vi "Cholesky Decomposition.vi"   [LabVIEW 2020]
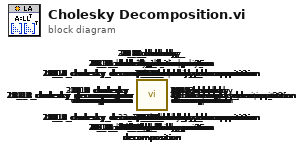
[diagram p0: block diagram]
diagram:
  n1 = call "32_16_cholesky_decomposition.vi"() -> ()  [unwired: 3 in, 1 out]
  n2 = call "32_15_cholesky_decomposition.vi"() -> ()  [unwired: 3 in, 1 out]
  n3 = call "32_14_cholesky_decomposition.vi"() -> ()  [unwired: 3 in, 1 out]
  n4 = call "32_13_cholesky_decomposition.vi"() -> ()  [unwired: 3 in, 1 out]
  n5 = call "32_12_cholesky_decomposition.vi"() -> ()  [unwired: 3 in, 1 out]
  n6 = call "32_11_cholesky_decomposition.vi"() -> ()  [unwired: 3 in, 1 out]
  n7 = call "32_10_cholesky_decomposition.vi"() -> ()  [unwired: 3 in, 1 out]
  n8 = call "32_9_cholesky_decomposition.vi"() -> ()  [unwired: 3 in, 1 out]
  n9 = call "32_8_cholesky_decomposition.vi"() -> ()  [unwired: 3 in, 1 out]
  n10 = call "32_7_cholesky_decomposition.vi"() -> ()  [unwired: 3 in, 1 out]
  n11 = call "32_6_cholesky_decomposition.vi"() -> ()  [unwired: 3 in, 1 out]
  n12 = call "32_5_cholesky_decomposition.vi"() -> ()  [unwired: 3 in, 1 out]
  n13 = call "32_4_cholesky_decomposition.vi"() -> ()  [unwired: 3 in, 1 out]
  n14 = call "32_3_cholesky_decomposition.vi"() -> ()  [unwired: 3 in, 1 out]
  n15 = call "32_2_cholesky_decomposition.vi"() -> ()  [unwired: 3 in, 1 out]
  n16 = call "32_1_cholesky_decomposition.vi"() -> ()  [unwired: 3 in, 1 out]
  n17 = call "31_16_cholesky_decomposition.vi"() -> ()  [unwired: 3 in, 1 out]
  n18 = call "31_15_cholesky_decomposition.vi"() -> ()  [unwired: 3 in, 1 out]
  n19 = call "31_14_cholesky_decomposition.vi"() -> ()  [unwired: 3 in, 1 out]
  n20 = call "31_13_cholesky_decomposition.vi"() -> ()  [unwired: 3 in, 1 out]
  n21 = call "31_12_cholesky_decomposition.vi"() -> ()  [unwired: 3 in, 1 out]
  n22 = call "31_11_cholesky_decomposition.vi"() -> ()  [unwired: 3 in, 1 out]
  n23 = call "31_10_cholesky_decomposition.vi"() -> ()  [unwired: 3 in, 1 out]
  n24 = call "31_9_cholesky_decomposition.vi"() -> ()  [unwired: 3 in, 1 out]
  n25 = call "31_8_cholesky_decomposition.vi"() -> ()  [unwired: 3 in, 1 out]
  n26 = call "31_7_cholesky_decomposition.vi"() -> ()  [unwired: 3 in, 1 out]
  n27 = call "31_6_cholesky_decomposition.vi"() -> ()  [unwired: 3 in, 1 out]
  n28 = call "31_5_cholesky_decomposition.vi"() -> ()  [unwired: 3 in, 1 out]
  n29 = call "31_4_cholesky_decomposition.vi"() -> ()  [unwired: 3 in, 1 out]
  n30 = call "31_3_cholesky_decomposition.vi"() -> ()  [unwired: 3 in, 1 out]
  n31 = call "31_2_cholesky_decomposition.vi"() -> ()  [unwired: 3 in, 1 out]
  n32 = call "31_1_cholesky_decomposition.vi"() -> ()  [unwired: 3 in, 1 out]
  n33 = call "30_16_cholesky_decomposition.vi"() -> ()  [unwired: 3 in, 1 out]
  n34 = call "30_15_cholesky_decomposition.vi"() -> ()  [unwired: 3 in, 1 out]
  n35 = call "30_14_cholesky_decomposition.vi"() -> ()  [unwired: 3 in, 1 out]
  n36 = call "30_13_cholesky_decomposition.vi"() -> ()  [unwired: 3 in, 1 out]
  n37 = call "30_12_cholesky_decomposition.vi"() -> ()  [unwired: 3 in, 1 out]
  n38 = call "30_11_cholesky_decomposition.vi"() -> ()  [unwired: 3 in, 1 out]
  n39 = call "30_10_cholesky_decomposition.vi"() -> ()  [unwired: 3 in, 1 out]
  n40 = call "30_9_cholesky_decomposition.vi"() -> ()  [unwired: 3 in, 1 out]
  n41 = call "30_8_cholesky_decomposition.vi"() -> ()  [unwired: 3 in, 1 out]
  n42 = call "30_7_cholesky_decomposition.vi"() -> ()  [unwired: 3 in, 1 out]
  n43 = call "30_6_cholesky_decomposition.vi"() -> ()  [unwired: 3 in, 1 out]
  n44 = call "30_5_cholesky_decomposition.vi"() -> ()  [unwired: 3 in, 1 out]
  n45 = call "30_4_cholesky_decomposition.vi"() -> ()  [unwired: 3 in, 1 out]
  n46 = call "30_3_cholesky_decomposition.vi"() -> ()  [unwired: 3 in, 1 out]
  n47 = call "30_2_cholesky_decomposition.vi"() -> ()  [unwired: 3 in, 1 out]
  n48 = call "30_1_cholesky_decomposition.vi"() -> ()  [unwired: 3 in, 1 out]
  n49 = call "29_16_cholesky_decomposition.vi"() -> ()  [unwired: 3 in, 1 out]
  n50 = call "29_15_cholesky_decomposition.vi"() -> ()  [unwired: 3 in, 1 out]
  n51 = call "29_14_cholesky_decomposition.vi"() -> ()  [unwired: 3 in, 1 out]
  n52 = call "29_13_cholesky_decomposition.vi"() -> ()  [unwired: 3 in, 1 out]
  n53 = call "29_12_cholesky_decomposition.vi"() -> ()  [unwired: 3 in, 1 out]
  n54 = call "29_11_cholesky_decomposition.vi"() -> ()  [unwired: 3 in, 1 out]
  n55 = call "29_10_cholesky_decomposition.vi"() -> ()  [unwired: 3 in, 1 out]
  n56 = call "29_9_cholesky_decomposition.vi"() -> ()  [unwired: 3 in, 1 out]
  n57 = call "29_8_cholesky_decomposition.vi"() -> ()  [unwired: 3 in, 1 out]
  n58 = call "29_7_cholesky_decomposition.vi"() -> ()  [unwired: 3 in, 1 out]
  n59 = call "29_6_cholesky_decomposition.vi"() -> ()  [unwired: 3 in, 1 out]
  n60 = call "29_5_cholesky_decomposition.vi"() -> ()  [unwired: 3 in, 1 out]
  n61 = call "29_4_cholesky_decomposition.vi"() -> ()  [unwired: 3 in, 1 out]
  n62 = call "29_3_cholesky_decomposition.vi"() -> ()  [unwired: 3 in, 1 out]
  n63 = call "29_2_cholesky_decomposition.vi"() -> ()  [unwired: 3 in, 1 out]
  n64 = call "29_1_cholesky_decomposition.vi"() -> ()  [unwired: 3 in, 1 out]
  n65 = call "28_16_cholesky_decomposition.vi"() -> ()  [unwired: 3 in, 1 out]
  n66 = call "28_15_cholesky_decomposition.vi"() -> ()  [unwired: 3 in, 1 out]
  n67 = call "28_14_cholesky_decomposition.vi"() -> ()  [unwired: 3 in, 1 out]
  n68 = call "28_13_cholesky_decomposition.vi"() -> ()  [unwired: 3 in, 1 out]
  n69 = call "28_12_cholesky_decomposition.vi"() -> ()  [unwired: 3 in, 1 out]
  n70 = call "28_11_cholesky_decomposition.vi"() -> ()  [unwired: 3 in, 1 out]
  n71 = call "28_10_cholesky_decomposition.vi"() -> ()  [unwired: 3 in, 1 out]
  n72 = call "28_9_cholesky_decomposition.vi"() -> ()  [unwired: 3 in, 1 out]
  n73 = call "28_8_cholesky_decomposition.vi"() -> ()  [unwired: 3 in, 1 out]
  n74 = call "28_7_cholesky_decomposition.vi"() -> ()  [unwired: 3 in, 1 out]
  n75 = call "28_6_cholesky_decomposition.vi"() -> ()  [unwired: 3 in, 1 out]
  n76 = call "28_5_cholesky_decomposition.vi"() -> ()  [unwired: 3 in, 1 out]
  n77 = call "28_4_cholesky_decomposition.vi"() -> ()  [unwired: 3 in, 1 out]
  n78 = call "28_3_cholesky_decomposition.vi"() -> ()  [unwired: 3 in, 1 out]
  n79 = call "28_2_cholesky_decomposition.vi"() -> ()  [unwired: 3 in, 1 out]
  n80 = call "28_1_cholesky_decomposition.vi"() -> ()  [unwired: 3 in, 1 out]
  n81 = call "27_16_cholesky_decomposition.vi"() -> ()  [unwired: 3 in, 1 out]
  n82 = call "27_15_cholesky_decomposition.vi"() -> ()  [unwired: 3 in, 1 out]
  n83 = call "27_14_cholesky_decomposition.vi"() -> ()  [unwired: 3 in, 1 out]
  n84 = call "27_13_cholesky_decomposition.vi"() -> ()  [unwired: 3 in, 1 out]
  n85 = call "27_12_cholesky_decomposition.vi"() -> ()  [unwired: 3 in, 1 out]
  n86 = call "27_11_cholesky_decomposition.vi"() -> ()  [unwired: 3 in, 1 out]
  n87 = call "27_10_cholesky_decomposition.vi"() -> ()  [unwired: 3 in, 1 out]
  n88 = call "27_9_cholesky_decomposition.vi"() -> ()  [unwired: 3 in, 1 out]
  n89 = call "27_8_cholesky_decomposition.vi"() -> ()  [unwired: 3 in, 1 out]
  n90 = call "27_7_cholesky_decomposition.vi"() -> ()  [unwired: 3 in, 1 out]
  n91 = call "27_6_cholesky_decomposition.vi"() -> ()  [unwired: 3 in, 1 out]
  n92 = call "27_5_cholesky_decomposition.vi"() -> ()  [unwired: 3 in, 1 out]
  n93 = call "27_4_cholesky_decomposition.vi"() -> ()  [unwired: 3 in, 1 out]
  n94 = call "27_3_cholesky_decomposition.vi"() -> ()  [unwired: 3 in, 1 out]
  n95 = call "27_2_cholesky_decomposition.vi"() -> ()  [unwired: 3 in, 1 out]
  n96 = call "27_1_cholesky_decomposition.vi"() -> ()  [unwired: 3 in, 1 out]
  n97 = call "26_16_cholesky_decomposition.vi"() -> ()  [unwired: 3 in, 1 out]
  n98 = call "26_15_cholesky_decomposition.vi"() -> ()  [unwired: 3 in, 1 out]
  n99 = call "26_14_cholesky_decomposition.vi"() -> ()  [unwired: 3 in, 1 out]
  n100 = call "26_13_cholesky_decomposition.vi"() -> ()  [unwired: 3 in, 1 out]
  n101 = call "26_12_cholesky_decomposition.vi"() -> ()  [unwired: 3 in, 1 out]
  n102 = call "26_11_cholesky_decomposition.vi"() -> ()  [unwired: 3 in, 1 out]
  n103 = call "26_10_cholesky_decomposition.vi"() -> ()  [unwired: 3 in, 1 out]
  n104 = call "26_9_cholesky_decomposition.vi"() -> ()  [unwired: 3 in, 1 out]
  n105 = call "26_8_cholesky_decomposition.vi"() -> ()  [unwired: 3 in, 1 out]
  n106 = call "26_7_cholesky_decomposition.vi"() -> ()  [unwired: 3 in, 1 out]
  n107 = call "26_6_cholesky_decomposition.vi"() -> ()  [unwired: 3 in, 1 out]
  n108 = call "26_5_cholesky_decomposition.vi"() -> ()  [unwired: 3 in, 1 out]
  n109 = call "26_4_cholesky_decomposition.vi"() -> ()  [unwired: 3 in, 1 out]
  n110 = call "26_3_cholesky_decomposition.vi"() -> ()  [unwired: 3 in, 1 out]
  n111 = call "26_2_cholesky_decomposition.vi"() -> ()  [unwired: 3 in, 1 out]
  n112 = call "26_1_cholesky_decomposition.vi"() -> ()  [unwired: 3 in, 1 out]
  n113 = call "25_16_cholesky_decomposition.vi"() -> ()  [unwired: 3 in, 1 out]
  n114 = call "25_15_cholesky_decomposition.vi"() -> ()  [unwired: 3 in, 1 out]
  n115 = call "25_14_cholesky_decomposition.vi"() -> ()  [unwired: 3 in, 1 out]
  n116 = call "25_13_cholesky_decomposition.vi"() -> ()  [unwired: 3 in, 1 out]
  n117 = call "25_12_cholesky_decomposition.vi"() -> ()  [unwired: 3 in, 1 out]
  n118 = call "25_11_cholesky_decomposition.vi"() -> ()  [unwired: 3 in, 1 out]
  n119 = call "25_10_cholesky_decomposition.vi"() -> ()  [unwired: 3 in, 1 out]
  n120 = call "25_9_cholesky_decomposition.vi"() -> ()  [unwired: 3 in, 1 out]
  n121 = call "25_8_cholesky_decomposition.vi"() -> ()  [unwired: 3 in, 1 out]
  n122 = call "25_7_cholesky_decomposition.vi"() -> ()  [unwired: 3 in, 1 out]
  n123 = call "25_6_cholesky_decomposition.vi"() -> ()  [unwired: 3 in, 1 out]
  n124 = call "25_5_cholesky_decomposition.vi"() -> ()  [unwired: 3 in, 1 out]
  n125 = call "25_4_cholesky_decomposition.vi"() -> ()  [unwired: 3 in, 1 out]
  n126 = call "25_3_cholesky_decomposition.vi"() -> ()  [unwired: 3 in, 1 out]
  n127 = call "25_2_cholesky_decomposition.vi"() -> ()  [unwired: 3 in, 1 out]
  n128 = call "25_1_cholesky_decomposition.vi"() -> ()  [unwired: 3 in, 1 out]
  n129 = call "24_16_cholesky_decomposition.vi"() -> ()  [unwired: 3 in, 1 out]
  n130 = call "24_15_cholesky_decomposition.vi"() -> ()  [unwired: 3 in, 1 out]
  n131 = call "24_14_cholesky_decomposition.vi"() -> ()  [unwired: 3 in, 1 out]
  n132 = call "24_13_cholesky_decomposition.vi"() -> ()  [unwired: 3 in, 1 out]
  n133 = call "24_12_cholesky_decomposition.vi"() -> ()  [unwired: 3 in, 1 out]
  n134 = call "24_11_cholesky_decomposition.vi"() -> ()  [unwired: 3 in, 1 out]
  n135 = call "24_10_cholesky_decomposition.vi"() -> ()  [unwired: 3 in, 1 out]
  n136 = call "24_9_cholesky_decomposition.vi"() -> ()  [unwired: 3 in, 1 out]
  n137 = call "24_8_cholesky_decomposition.vi"() -> ()  [unwired: 3 in, 1 out]
  n138 = call "24_7_cholesky_decomposition.vi"() -> ()  [unwired: 3 in, 1 out]
  n139 = call "24_6_cholesky_decomposition.vi"() -> ()  [unwired: 3 in, 1 out]
  n140 = call "24_5_cholesky_decomposition.vi"() -> ()  [unwired: 3 in, 1 out]
  n141 = call "24_4_cholesky_decomposition.vi"() -> ()  [unwired: 3 in, 1 out]
  n142 = call "24_3_cholesky_decomposition.vi"() -> ()  [unwired: 3 in, 1 out]
  n143 = call "24_2_cholesky_decomposition.vi"() -> ()  [unwired: 3 in, 1 out]
  n144 = call "24_1_cholesky_decomposition.vi"() -> ()  [unwired: 3 in, 1 out]
  n145 = call "23_16_cholesky_decomposition.vi"() -> ()  [unwired: 3 in, 1 out]
  n146 = call "23_15_cholesky_decomposition.vi"() -> ()  [unwired: 3 in, 1 out]
  n147 = call "23_14_cholesky_decomposition.vi"() -> ()  [unwired: 3 in, 1 out]
  n148 = call "23_13_cholesky_decomposition.vi"() -> ()  [unwired: 3 in, 1 out]
  n149 = call "23_12_cholesky_decomposition.vi"() -> ()  [unwired: 3 in, 1 out]
  n150 = call "23_11_cholesky_decomposition.vi"() -> ()  [unwired: 3 in, 1 out]
  n151 = call "23_10_cholesky_decomposition.vi"() -> ()  [unwired: 3 in, 1 out]
  n152 = call "23_9_cholesky_decomposition.vi"() -> ()  [unwired: 3 in, 1 out]
  n153 = call "23_8_cholesky_decomposition.vi"() -> ()  [unwired: 3 in, 1 out]
  n154 = call "23_7_cholesky_decomposition.vi"() -> ()  [unwired: 3 in, 1 out]
  n155 = call "23_6_cholesky_decomposition.vi"() -> ()  [unwired: 3 in, 1 out]
  n156 = call "23_5_cholesky_decomposition.vi"() -> ()  [unwired: 3 in, 1 out]
  n157 = call "23_4_cholesky_decomposition.vi"() -> ()  [unwired: 3 in, 1 out]
  n158 = call "23_3_cholesky_decomposition.vi"() -> ()  [unwired: 3 in, 1 out]
  n159 = call "23_2_cholesky_decomposition.vi"() -> ()  [unwired: 3 in, 1 out]
  n160 = call "23_1_cholesky_decomposition.vi"() -> ()  [unwired: 3 in, 1 out]
  n161 = call "22_16_cholesky_decomposition.vi"() -> ()  [unwired: 3 in, 1 out]
  n162 = call "22_15_cholesky_decomposition.vi"() -> ()  [unwired: 3 in, 1 out]
  n163 = call "22_14_cholesky_decomposition.vi"() -> ()  [unwired: 3 in, 1 out]
  n164 = call "22_13_cholesky_decomposition.vi"() -> ()  [unwired: 3 in, 1 out]
  n165 = call "22_12_cholesky_decomposition.vi"() -> ()  [unwired: 3 in, 1 out]
  n166 = call "22_11_cholesky_decomposition.vi"() -> ()  [unwired: 3 in, 1 out]
  n167 = call "22_10_cholesky_decomposition.vi"() -> ()  [unwired: 3 in, 1 out]
  n168 = call "22_9_cholesky_decomposition.vi"() -> ()  [unwired: 3 in, 1 out]
  n169 = call "22_8_cholesky_decomposition.vi"() -> ()  [unwired: 3 in, 1 out]
  n170 = call "22_7_cholesky_decomposition.vi"() -> ()  [unwired: 3 in, 1 out]
  n171 = call "22_6_cholesky_decomposition.vi"() -> ()  [unwired: 3 in, 1 out]
  n172 = call "22_5_cholesky_decomposition.vi"() -> ()  [unwired: 3 in, 1 out]
  n173 = call "22_4_cholesky_decomposition.vi"() -> ()  [unwired: 3 in, 1 out]
  n174 = call "22_3_cholesky_decomposition.vi"() -> ()  [unwired: 3 in, 1 out]
  n175 = call "22_2_cholesky_decomposition.vi"() -> ()  [unwired: 3 in, 1 out]
  n176 = call "22_1_cholesky_decomposition.vi"() -> ()  [unwired: 3 in, 1 out]
  n177 = call "21_16_cholesky_decomposition.vi"() -> ()  [unwired: 3 in, 1 out]
  n178 = call "21_15_cholesky_decomposition.vi"() -> ()  [unwired: 3 in, 1 out]
  n179 = call "21_14_cholesky_decomposition.vi"() -> ()  [unwired: 3 in, 1 out]
  n180 = call "21_13_cholesky_decomposition.vi"() -> ()  [unwired: 3 in, 1 out]
  n181 = call "21_12_cholesky_decomposition.vi"() -> ()  [unwired: 3 in, 1 out]
  n182 = call "21_11_cholesky_decomposition.vi"() -> ()  [unwired: 3 in, 1 out]
  n183 = call "21_10_cholesky_decomposition.vi"() -> ()  [unwired: 3 in, 1 out]
  n184 = call "21_9_cholesky_decomposition.vi"() -> ()  [unwired: 3 in, 1 out]
  n185 = call "21_8_cholesky_decomposition.vi"() -> ()  [unwired: 3 in, 1 out]
  n186 = call "21_7_cholesky_decomposition.vi"() -> ()  [unwired: 3 in, 1 out]
  n187 = call "21_6_cholesky_decomposition.vi"() -> ()  [unwired: 3 in, 1 out]
  n188 = call "21_5_cholesky_decomposition.vi"() -> ()  [unwired: 3 in, 1 out]
  n189 = call "21_4_cholesky_decomposition.vi"() -> ()  [unwired: 3 in, 1 out]
  n190 = call "21_3_cholesky_decomposition.vi"() -> ()  [unwired: 3 in, 1 out]
  n191 = call "21_2_cholesky_decomposition.vi"() -> ()  [unwired: 3 in, 1 out]
  n192 = call "21_1_cholesky_decomposition.vi"() -> ()  [unwired: 3 in, 1 out]
  n193 = call "20_16_cholesky_decomposition.vi"() -> ()  [unwired: 3 in, 1 out]
  n194 = call "20_15_cholesky_decomposition.vi"() -> ()  [unwired: 3 in, 1 out]
  n195 = call "20_14_cholesky_decomposition.vi"() -> ()  [unwired: 3 in, 1 out]
  n196 = call "20_13_cholesky_decomposition.vi"() -> ()  [unwired: 3 in, 1 out]
  n197 = call "20_12_cholesky_decomposition.vi"() -> ()  [unwired: 3 in, 1 out]
  n198 = call "20_11_cholesky_decomposition.vi"() -> ()  [unwired: 3 in, 1 out]
  n199 = call "20_10_cholesky_decomposition.vi"() -> ()  [unwired: 3 in, 1 out]
  n200 = call "20_9_cholesky_decomposition.vi"() -> ()  [unwired: 3 in, 1 out]
  n201 = call "20_8_cholesky_decomposition.vi"() -> ()  [unwired: 3 in, 1 out]
  n202 = call "20_7_cholesky_decomposition.vi"() -> ()  [unwired: 3 in, 1 out]
  n203 = call "20_6_cholesky_decomposition.vi"() -> ()  [unwired: 3 in, 1 out]
  n204 = call "20_5_cholesky_decomposition.vi"() -> ()  [unwired: 3 in, 1 out]
  n205 = call "20_4_cholesky_decomposition.vi"() -> ()  [unwired: 3 in, 1 out]
  n206 = call "20_3_cholesky_decomposition.vi"() -> ()  [unwired: 3 in, 1 out]
  n207 = call "20_2_cholesky_decomposition.vi"() -> ()  [unwired: 3 in, 1 out]
  n208 = call "20_1_cholesky_decomposition.vi"() -> ()  [unwired: 3 in, 1 out]
  n209 = call "19_16_cholesky_decomposition.vi"() -> ()  [unwired: 3 in, 1 out]
  n210 = call "19_15_cholesky_decomposition.vi"() -> ()  [unwired: 3 in, 1 out]
  n211 = call "19_14_cholesky_decomposition.vi"() -> ()  [unwired: 3 in, 1 out]
  n212 = call "19_13_cholesky_decomposition.vi"() -> ()  [unwired: 3 in, 1 out]
  n213 = call "19_12_cholesky_decomposition.vi"() -> ()  [unwired: 3 in, 1 out]
  n214 = call "19_11_cholesky_decomposition.vi"() -> ()  [unwired: 3 in, 1 out]
  n215 = call "19_10_cholesky_decomposition.vi"() -> ()  [unwired: 3 in, 1 out]
  n216 = call "19_9_cholesky_decomposition.vi"() -> ()  [unwired: 3 in, 1 out]
  n217 = call "19_8_cholesky_decomposition.vi"() -> ()  [unwired: 3 in, 1 out]
  n218 = call "19_7_cholesky_decomposition.vi"() -> ()  [unwired: 3 in, 1 out]
  n219 = call "19_6_cholesky_decomposition.vi"() -> ()  [unwired: 3 in, 1 out]
  n220 = call "19_5_cholesky_decomposition.vi"() -> ()  [unwired: 3 in, 1 out]
  n221 = call "19_4_cholesky_decomposition.vi"() -> ()  [unwired: 3 in, 1 out]
  n222 = call "19_3_cholesky_decomposition.vi"() -> ()  [unwired: 3 in, 1 out]
  n223 = call "19_2_cholesky_decomposition.vi"() -> ()  [unwired: 3 in, 1 out]
  n224 = call "19_1_cholesky_decomposition.vi"() -> ()  [unwired: 3 in, 1 out]
  n225 = call "18_16_cholesky_decomposition.vi"() -> ()  [unwired: 3 in, 1 out]
  n226 = call "18_15_cholesky_decomposition.vi"() -> ()  [unwired: 3 in, 1 out]
  n227 = call "18_14_cholesky_decomposition.vi"() -> ()  [unwired: 3 in, 1 out]
  n228 = call "18_13_cholesky_decomposition.vi"() -> ()  [unwired: 3 in, 1 out]
  n229 = call "18_12_cholesky_decomposition.vi"() -> ()  [unwired: 3 in, 1 out]
  n230 = call "18_11_cholesky_decomposition.vi"() -> ()  [unwired: 3 in, 1 out]
  n231 = call "18_10_cholesky_decomposition.vi"() -> ()  [unwired: 3 in, 1 out]
  n232 = call "18_9_cholesky_decomposition.vi"() -> ()  [unwired: 3 in, 1 out]
  n233 = call "18_8_cholesky_decomposition.vi"() -> ()  [unwired: 3 in, 1 out]
  n234 = call "18_7_cholesky_decomposition.vi"() -> ()  [unwired: 3 in, 1 out]
  n235 = call "18_6_cholesky_decomposition.vi"() -> ()  [unwired: 3 in, 1 out]
  n236 = call "18_5_cholesky_decomposition.vi"() -> ()  [unwired: 3 in, 1 out]
  n237 = call "18_4_cholesky_decomposition.vi"() -> ()  [unwired: 3 in, 1 out]
  n238 = call "18_3_cholesky_decomposition.vi"() -> ()  [unwired: 3 in, 1 out]
  n239 = call "18_2_cholesky_decomposition.vi"() -> ()  [unwired: 3 in, 1 out]
  n240 = call "18_1_cholesky_decomposition.vi"() -> ()  [unwired: 3 in, 1 out]
  n241 = call "17_16_cholesky_decomposition.vi"() -> ()  [unwired: 3 in, 1 out]
  n242 = call "17_15_cholesky_decomposition.vi"() -> ()  [unwired: 3 in, 1 out]
  n243 = call "17_14_cholesky_decomposition.vi"() -> ()  [unwired: 3 in, 1 out]
  n244 = call "17_13_cholesky_decomposition.vi"() -> ()  [unwired: 3 in, 1 out]
  n245 = call "17_12_cholesky_decomposition.vi"() -> ()  [unwired: 3 in, 1 out]
  n246 = call "17_11_cholesky_decomposition.vi"() -> ()  [unwired: 3 in, 1 out]
  n247 = call "17_10_cholesky_decomposition.vi"() -> ()  [unwired: 3 in, 1 out]
  n248 = call "17_9_cholesky_decomposition.vi"() -> ()  [unwired: 3 in, 1 out]
  n249 = call "17_8_cholesky_decomposition.vi"() -> ()  [unwired: 3 in, 1 out]
  n250 = call "17_7_cholesky_decomposition.vi"() -> ()  [unwired: 3 in, 1 out]
  n251 = call "17_6_cholesky_decomposition.vi"() -> ()  [unwired: 3 in, 1 out]
  n252 = call "17_5_cholesky_decomposition.vi"() -> ()  [unwired: 3 in, 1 out]
  n253 = call "17_4_cholesky_decomposition.vi"() -> ()  [unwired: 3 in, 1 out]
  n254 = call "17_3_cholesky_decomposition.vi"() -> ()  [unwired: 3 in, 1 out]
  n255 = call "17_2_cholesky_decomposition.vi"() -> ()  [unwired: 3 in, 1 out]
  n256 = call "17_1_cholesky_decomposition.vi"() -> ()  [unwired: 3 in, 1 out]
  n257 = call "16_16_cholesky_decomposition.vi"() -> ()  [unwired: 3 in, 1 out]
  n258 = call "16_15_cholesky_decomposition.vi"() -> ()  [unwired: 3 in, 1 out]
  n259 = call "16_14_cholesky_decomposition.vi"() -> ()  [unwired: 3 in, 1 out]
  n260 = call "16_13_cholesky_decomposition.vi"() -> ()  [unwired: 3 in, 1 out]
  n261 = call "16_12_cholesky_decomposition.vi"() -> ()  [unwired: 3 in, 1 out]
  n262 = call "16_11_cholesky_decomposition.vi"() -> ()  [unwired: 3 in, 1 out]
  n263 = call "16_10_cholesky_decomposition.vi"() -> ()  [unwired: 3 in, 1 out]
  n264 = call "16_9_cholesky_decomposition.vi"() -> ()  [unwired: 3 in, 1 out]
  n265 = call "16_8_cholesky_decomposition.vi"() -> ()  [unwired: 3 in, 1 out]
  n266 = call "16_7_cholesky_decomposition.vi"() -> ()  [unwired: 3 in, 1 out]
  n267 = call "16_6_cholesky_decomposition.vi"() -> ()  [unwired: 3 in, 1 out]
  n268 = call "16_5_cholesky_decomposition.vi"() -> ()  [unwired: 3 in, 1 out]
  n269 = call "16_4_cholesky_decomposition.vi"() -> ()  [unwired: 3 in, 1 out]
  n270 = call "16_3_cholesky_decomposition.vi"() -> ()  [unwired: 3 in, 1 out]
  n271 = call "16_2_cholesky_decomposition.vi"() -> ()  [unwired: 3 in, 1 out]
  n272 = call "16_1_cholesky_decomposition.vi"() -> ()  [unwired: 3 in, 1 out]
  n273 = call "15_16_cholesky_decomposition.vi"() -> ()  [unwired: 3 in, 1 out]
  n274 = call "15_15_cholesky_decomposition.vi"() -> ()  [unwired: 3 in, 1 out]
  n275 = call "15_14_cholesky_decomposition.vi"() -> ()  [unwired: 3 in, 1 out]
  n276 = call "15_13_cholesky_decomposition.vi"() -> ()  [unwired: 3 in, 1 out]
  n277 = call "15_12_cholesky_decomposition.vi"() -> ()  [unwired: 3 in, 1 out]
  n278 = call "15_11_cholesky_decomposition.vi"() -> ()  [unwired: 3 in, 1 out]
  n279 = call "15_10_cholesky_decomposition.vi"() -> ()  [unwired: 3 in, 1 out]
  n280 = call "15_9_cholesky_decomposition.vi"() -> ()  [unwired: 3 in, 1 out]
  n281 = call "15_8_cholesky_decomposition.vi"() -> ()  [unwired: 3 in, 1 out]
  n282 = call "15_7_cholesky_decomposition.vi"() -> ()  [unwired: 3 in, 1 out]
  n283 = call "15_6_cholesky_decomposition.vi"() -> ()  [unwired: 3 in, 1 out]
  n284 = call "15_5_cholesky_decomposition.vi"() -> ()  [unwired: 3 in, 1 out]
  n285 = call "15_4_cholesky_decomposition.vi"() -> ()  [unwired: 3 in, 1 out]
  n286 = call "15_3_cholesky_decomposition.vi"() -> ()  [unwired: 3 in, 1 out]
  n287 = call "15_2_cholesky_decomposition.vi"() -> ()  [unwired: 3 in, 1 out]
  n288 = call "15_1_cholesky_decomposition.vi"() -> ()  [unwired: 3 in, 1 out]
  n289 = call "14_16_cholesky_decomposition.vi"() -> ()  [unwired: 3 in, 1 out]
  n290 = call "14_15_cholesky_decomposition.vi"() -> ()  [unwired: 3 in, 1 out]
  n291 = call "14_14_cholesky_decomposition.vi"() -> ()  [unwired: 3 in, 1 out]
  n292 = call "14_13_cholesky_decomposition.vi"() -> ()  [unwired: 3 in, 1 out]
  n293 = call "14_12_cholesky_decomposition.vi"() -> ()  [unwired: 3 in, 1 out]
  n294 = call "14_11_cholesky_decomposition.vi"() -> ()  [unwired: 3 in, 1 out]
  n295 = call "14_10_cholesky_decomposition.vi"() -> ()  [unwired: 3 in, 1 out]
  n296 = call "14_9_cholesky_decomposition.vi"() -> ()  [unwired: 3 in, 1 out]
  n297 = call "14_8_cholesky_decomposition.vi"() -> ()  [unwired: 3 in, 1 out]
  n298 = call "14_7_cholesky_decomposition.vi"() -> ()  [unwired: 3 in, 1 out]
  n299 = call "14_6_cholesky_decomposition.vi"() -> ()  [unwired: 3 in, 1 out]
  n300 = call "14_5_cholesky_decomposition.vi"() -> ()  [unwired: 3 in, 1 out]
  n301 = call "14_4_cholesky_decomposition.vi"() -> ()  [unwired: 3 in, 1 out]
  n302 = call "14_3_cholesky_decomposition.vi"() -> ()  [unwired: 3 in, 1 out]
  n303 = call "14_2_cholesky_decomposition.vi"() -> ()  [unwired: 3 in, 1 out]
  n304 = call "14_1_cholesky_decomposition.vi"() -> ()  [unwired: 3 in, 1 out]
  n305 = call "13_16_cholesky_decomposition.vi"() -> ()  [unwired: 3 in, 1 out]
  n306 = call "13_15_cholesky_decomposition.vi"() -> ()  [unwired: 3 in, 1 out]
  n307 = call "13_14_cholesky_decomposition.vi"() -> ()  [unwired: 3 in, 1 out]
  n308 = call "13_13_cholesky_decomposition.vi"() -> ()  [unwired: 3 in, 1 out]
  n309 = call "13_12_cholesky_decomposition.vi"() -> ()  [unwired: 3 in, 1 out]
  n310 = call "13_11_cholesky_decomposition.vi"() -> ()  [unwired: 3 in, 1 out]
  n311 = call "13_10_cholesky_decomposition.vi"() -> ()  [unwired: 3 in, 1 out]
  n312 = call "13_9_cholesky_decomposition.vi"() -> ()  [unwired: 3 in, 1 out]
  n313 = call "13_8_cholesky_decomposition.vi"() -> ()  [unwired: 3 in, 1 out]
  n314 = call "13_7_cholesky_decomposition.vi"() -> ()  [unwired: 3 in, 1 out]
  n315 = call "13_6_cholesky_decomposition.vi"() -> ()  [unwired: 3 in, 1 out]
  n316 = call "13_5_cholesky_decomposition.vi"() -> ()  [unwired: 3 in, 1 out]
  n317 = call "13_4_cholesky_decomposition.vi"() -> ()  [unwired: 3 in, 1 out]
  n318 = call "13_3_cholesky_decomposition.vi"() -> ()  [unwired: 3 in, 1 out]
  n319 = call "13_2_cholesky_decomposition.vi"() -> ()  [unwired: 3 in, 1 out]
  n320 = call "13_1_cholesky_decomposition.vi"() -> ()  [unwired: 3 in, 1 out]
  n321 = call "12_16_cholesky_decomposition.vi"() -> ()  [unwired: 3 in, 1 out]
  n322 = call "12_15_cholesky_decomposition.vi"() -> ()  [unwired: 3 in, 1 out]
  n323 = call "12_14_cholesky_decomposition.vi"() -> ()  [unwired: 3 in, 1 out]
  n324 = call "12_13_cholesky_decomposition.vi"() -> ()  [unwired: 3 in, 1 out]
  n325 = call "12_12_cholesky_decomposition.vi"() -> ()  [unwired: 3 in, 1 out]
  n326 = call "12_11_cholesky_decomposition.vi"() -> ()  [unwired: 3 in, 1 out]
  n327 = call "12_10_cholesky_decomposition.vi"() -> ()  [unwired: 3 in, 1 out]
  n328 = call "12_9_cholesky_decomposition.vi"() -> ()  [unwired: 3 in, 1 out]
  n329 = call "12_8_cholesky_decomposition.vi"() -> ()  [unwired: 3 in, 1 out]
  n330 = call "12_7_cholesky_decomposition.vi"() -> ()  [unwired: 3 in, 1 out]
  n331 = call "12_6_cholesky_decomposition.vi"() -> ()  [unwired: 3 in, 1 out]
  n332 = call "12_5_cholesky_decomposition.vi"() -> ()  [unwired: 3 in, 1 out]
  n333 = call "12_4_cholesky_decomposition.vi"() -> ()  [unwired: 3 in, 1 out]
  n334 = call "12_3_cholesky_decomposition.vi"() -> ()  [unwired: 3 in, 1 out]
  n335 = call "12_2_cholesky_decomposition.vi"() -> ()  [unwired: 3 in, 1 out]
  n336 = call "12_1_cholesky_decomposition.vi"() -> ()  [unwired: 3 in, 1 out]
  n337 = call "11_16_cholesky_decomposition.vi"() -> ()  [unwired: 3 in, 1 out]
  n338 = call "11_15_cholesky_decomposition.vi"() -> ()  [unwired: 3 in, 1 out]
  n339 = call "11_14_cholesky_decomposition.vi"() -> ()  [unwired: 3 in, 1 out]
  n340 = call "11_13_cholesky_decomposition.vi"() -> ()  [unwired: 3 in, 1 out]
  n341 = call "11_12_cholesky_decomposition.vi"() -> ()  [unwired: 3 in, 1 out]
  n342 = call "11_11_cholesky_decomposition.vi"() -> ()  [unwired: 3 in, 1 out]
  n343 = call "11_10_cholesky_decomposition.vi"() -> ()  [unwired: 3 in, 1 out]
  n344 = call "11_9_cholesky_decomposition.vi"() -> ()  [unwired: 3 in, 1 out]
  n345 = call "11_8_cholesky_decomposition.vi"() -> ()  [unwired: 3 in, 1 out]
  n346 = call "11_7_cholesky_decomposition.vi"() -> ()  [unwired: 3 in, 1 out]
  n347 = call "11_6_cholesky_decomposition.vi"() -> ()  [unwired: 3 in, 1 out]
  n348 = call "11_5_cholesky_decomposition.vi"() -> ()  [unwired: 3 in, 1 out]
  n349 = call "11_4_cholesky_decomposition.vi"() -> ()  [unwired: 3 in, 1 out]
  n350 = call "11_3_cholesky_decomposition.vi"() -> ()  [unwired: 3 in, 1 out]
  n351 = call "11_2_cholesky_decomposition.vi"() -> ()  [unwired: 3 in, 1 out]
  n352 = call "11_1_cholesky_decomposition.vi"() -> ()  [unwired: 3 in, 1 out]
  n353 = call "10_16_cholesky_decomposition.vi"() -> ()  [unwired: 3 in, 1 out]
  n354 = call "10_15_cholesky_decomposition.vi"() -> ()  [unwired: 3 in, 1 out]
  n355 = call "10_14_cholesky_decomposition.vi"() -> ()  [unwired: 3 in, 1 out]
  n356 = call "10_13_cholesky_decomposition.vi"() -> ()  [unwired: 3 in, 1 out]
  n357 = call "10_12_cholesky_decomposition.vi"() -> ()  [unwired: 3 in, 1 out]
  n358 = call "10_11_cholesky_decomposition.vi"() -> ()  [unwired: 3 in, 1 out]
  n359 = call "10_10_cholesky_decomposition.vi"() -> ()  [unwired: 3 in, 1 out]
  n360 = call "10_9_cholesky_decomposition.vi"() -> ()  [unwired: 3 in, 1 out]
  n361 = call "10_8_cholesky_decomposition.vi"() -> ()  [unwired: 3 in, 1 out]
  n362 = call "10_7_cholesky_decomposition.vi"() -> ()  [unwired: 3 in, 1 out]
  n363 = call "10_6_cholesky_decomposition.vi"() -> ()  [unwired: 3 in, 1 out]
  n364 = call "10_5_cholesky_decomposition.vi"() -> ()  [unwired: 3 in, 1 out]
  n365 = call "10_4_cholesky_decomposition.vi"() -> ()  [unwired: 3 in, 1 out]
  n366 = call "10_3_cholesky_decomposition.vi"() -> ()  [unwired: 3 in, 1 out]
  n367 = call "10_2_cholesky_decomposition.vi"() -> ()  [unwired: 3 in, 1 out]
  n368 = call "10_1_cholesky_decomposition.vi"() -> ()  [unwired: 3 in, 1 out]
  n369 = call "9_16_cholesky_decomposition.vi"() -> ()  [unwired: 3 in, 1 out]
  n370 = call "9_15_cholesky_decomposition.vi"() -> ()  [unwired: 3 in, 1 out]
  n371 = call "9_14_cholesky_decomposition.vi"() -> ()  [unwired: 3 in, 1 out]
  n372 = call "9_13_cholesky_decomposition.vi"() -> ()  [unwired: 3 in, 1 out]
  n373 = call "9_12_cholesky_decomposition.vi"() -> ()  [unwired: 3 in, 1 out]
  n374 = call "9_11_cholesky_decomposition.vi"() -> ()  [unwired: 3 in, 1 out]
  n375 = call "9_10_cholesky_decomposition.vi"() -> ()  [unwired: 3 in, 1 out]
  n376 = call "9_9_cholesky_decomposition.vi"() -> ()  [unwired: 3 in, 1 out]
  n377 = call "9_8_cholesky_decomposition.vi"() -> ()  [unwired: 3 in, 1 out]
  n378 = call "9_7_cholesky_decomposition.vi"() -> ()  [unwired: 3 in, 1 out]
  n379 = call "9_6_cholesky_decomposition.vi"() -> ()  [unwired: 3 in, 1 out]
  n380 = call "9_5_cholesky_decomposition.vi"() -> ()  [unwired: 3 in, 1 out]
  n381 = call "9_4_cholesky_decomposition.vi"() -> ()  [unwired: 3 in, 1 out]
  n382 = call "9_3_cholesky_decomposition.vi"() -> ()  [unwired: 3 in, 1 out]
  n383 = call "9_2_cholesky_decomposition.vi"() -> ()  [unwired: 3 in, 1 out]
  n384 = call "9_1_cholesky_decomposition.vi"() -> ()  [unwired: 3 in, 1 out]
  n385 = call "8_16_cholesky_decomposition.vi"() -> ()  [unwired: 3 in, 1 out]
  n386 = call "8_15_cholesky_decomposition.vi"() -> ()  [unwired: 3 in, 1 out]
  n387 = call "8_14_cholesky_decomposition.vi"() -> ()  [unwired: 3 in, 1 out]
  n388 = call "8_13_cholesky_decomposition.vi"() -> ()  [unwired: 3 in, 1 out]
  n389 = call "8_12_cholesky_decomposition.vi"() -> ()  [unwired: 3 in, 1 out]
  n390 = call "8_11_cholesky_decomposition.vi"() -> ()  [unwired: 3 in, 1 out]
  n391 = call "8_10_cholesky_decomposition.vi"() -> ()  [unwired: 3 in, 1 out]
  n392 = call "8_9_cholesky_decomposition.vi"() -> ()  [unwired: 3 in, 1 out]
  n393 = call "8_8_cholesky_decomposition.vi"() -> ()  [unwired: 3 in, 1 out]
  n394 = call "8_7_cholesky_decomposition.vi"() -> ()  [unwired: 3 in, 1 out]
  n395 = call "8_6_cholesky_decomposition.vi"() -> ()  [unwired: 3 in, 1 out]
  n396 = call "8_5_cholesky_decomposition.vi"() -> ()  [unwired: 3 in, 1 out]
  n397 = call "8_4_cholesky_decomposition.vi"() -> ()  [unwired: 3 in, 1 out]
  n398 = call "8_3_cholesky_decomposition.vi"() -> ()  [unwired: 3 in, 1 out]
  n399 = call "8_2_cholesky_decomposition.vi"() -> ()  [unwired: 3 in, 1 out]
  n400 = call "8_1_cholesky_decomposition.vi"() -> ()  [unwired: 3 in, 1 out]
  n401 = call "7_16_cholesky_decomposition.vi"() -> ()  [unwired: 3 in, 1 out]
  n402 = call "7_15_cholesky_decomposition.vi"() -> ()  [unwired: 3 in, 1 out]
  n403 = call "7_14_cholesky_decomposition.vi"() -> ()  [unwired: 3 in, 1 out]
  n404 = call "7_13_cholesky_decomposition.vi"() -> ()  [unwired: 3 in, 1 out]
  n405 = call "7_12_cholesky_decomposition.vi"() -> ()  [unwired: 3 in, 1 out]
  n406 = call "7_11_cholesky_decomposition.vi"() -> ()  [unwired: 3 in, 1 out]
  n407 = call "7_10_cholesky_decomposition.vi"() -> ()  [unwired: 3 in, 1 out]
  n408 = call "7_9_cholesky_decomposition.vi"() -> ()  [unwired: 3 in, 1 out]
  n409 = call "7_8_cholesky_decomposition.vi"() -> ()  [unwired: 3 in, 1 out]
  n410 = call "7_7_cholesky_decomposition.vi"() -> ()  [unwired: 3 in, 1 out]
  n411 = call "7_6_cholesky_decomposition.vi"() -> ()  [unwired: 3 in, 1 out]
  n412 = call "7_5_cholesky_decomposition.vi"() -> ()  [unwired: 3 in, 1 out]
  n413 = call "7_4_cholesky_decomposition.vi"() -> ()  [unwired: 3 in, 1 out]
  n414 = call "7_3_cholesky_decomposition.vi"() -> ()  [unwired: 3 in, 1 out]
  n415 = call "7_2_cholesky_decomposition.vi"() -> ()  [unwired: 3 in, 1 out]
  n416 = call "7_1_cholesky_decomposition.vi"() -> ()  [unwired: 3 in, 1 out]
  n417 = call "6_16_cholesky_decomposition.vi"() -> ()  [unwired: 3 in, 1 out]
  n418 = call "6_15_cholesky_decomposition.vi"() -> ()  [unwired: 3 in, 1 out]
  n419 = call "6_14_cholesky_decomposition.vi"() -> ()  [unwired: 3 in, 1 out]
  n420 = call "6_13_cholesky_decomposition.vi"() -> ()  [unwired: 3 in, 1 out]
  n421 = call "6_12_cholesky_decomposition.vi"() -> ()  [unwired: 3 in, 1 out]
  n422 = call "6_11_cholesky_decomposition.vi"() -> ()  [unwired: 3 in, 1 out]
  n423 = call "6_10_cholesky_decomposition.vi"() -> ()  [unwired: 3 in, 1 out]
  n424 = call "6_9_cholesky_decomposition.vi"() -> ()  [unwired: 3 in, 1 out]
  n425 = call "6_8_cholesky_decomposition.vi"() -> ()  [unwired: 3 in, 1 out]
  n426 = call "6_7_cholesky_decomposition.vi"() -> ()  [unwired: 3 in, 1 out]
  n427 = call "6_6_cholesky_decomposition.vi"() -> ()  [unwired: 3 in, 1 out]
  n428 = call "6_5_cholesky_decomposition.vi"() -> ()  [unwired: 3 in, 1 out]
  n429 = call "6_4_cholesky_decomposition.vi"() -> ()  [unwired: 3 in, 1 out]
  n430 = call "6_3_cholesky_decomposition.vi"() -> ()  [unwired: 3 in, 1 out]
  n431 = call "6_2_cholesky_decomposition.vi"() -> ()  [unwired: 3 in, 1 out]
  n432 = call "6_1_cholesky_decomposition.vi"() -> ()  [unwired: 3 in, 1 out]
  n433 = call "5_16_cholesky_decomposition.vi"() -> ()  [unwired: 3 in, 1 out]
  n434 = call "5_15_cholesky_decomposition.vi"() -> ()  [unwired: 3 in, 1 out]
  n435 = call "5_14_cholesky_decomposition.vi"() -> ()  [unwired: 3 in, 1 out]
  n436 = call "5_13_cholesky_decomposition.vi"() -> ()  [unwired: 3 in, 1 out]
  n437 = call "5_12_cholesky_decomposition.vi"() -> ()  [unwired: 3 in, 1 out]
  n438 = call "5_11_cholesky_decomposition.vi"() -> ()  [unwired: 3 in, 1 out]
  n439 = call "5_10_cholesky_decomposition.vi"() -> ()  [unwired: 3 in, 1 out]
  n440 = call "5_9_cholesky_decomposition.vi"() -> ()  [unwired: 3 in, 1 out]
  n441 = call "5_8_cholesky_decomposition.vi"() -> ()  [unwired: 3 in, 1 out]
  n442 = call "5_7_cholesky_decomposition.vi"() -> ()  [unwired: 3 in, 1 out]
  n443 = call "5_6_cholesky_decomposition.vi"() -> ()  [unwired: 3 in, 1 out]
  n444 = call "5_5_cholesky_decomposition.vi"() -> ()  [unwired: 3 in, 1 out]
  n445 = call "5_4_cholesky_decomposition.vi"() -> ()  [unwired: 3 in, 1 out]
  n446 = call "5_3_cholesky_decomposition.vi"() -> ()  [unwired: 3 in, 1 out]
  n447 = call "5_2_cholesky_decomposition.vi"() -> ()  [unwired: 3 in, 1 out]
  n448 = call "5_1_cholesky_decomposition.vi"() -> ()  [unwired: 3 in, 1 out]
  n449 = call "4_16_cholesky_decomposition.vi"() -> ()  [unwired: 3 in, 1 out]
  n450 = call "4_15_cholesky_decomposition.vi"() -> ()  [unwired: 3 in, 1 out]
  n451 = call "4_14_cholesky_decomposition.vi"() -> ()  [unwired: 3 in, 1 out]
  n452 = call "4_13_cholesky_decomposition.vi"() -> ()  [unwired: 3 in, 1 out]
  n453 = call "4_12_cholesky_decomposition.vi"() -> ()  [unwired: 3 in, 1 out]
  n454 = call "4_11_cholesky_decomposition.vi"() -> ()  [unwired: 3 in, 1 out]
  n455 = call "4_10_cholesky_decomposition.vi"() -> ()  [unwired: 3 in, 1 out]
  n456 = call "4_9_cholesky_decomposition.vi"() -> ()  [unwired: 3 in, 1 out]
  n457 = call "4_8_cholesky_decomposition.vi"() -> ()  [unwired: 3 in, 1 out]
  n458 = call "4_7_cholesky_decomposition.vi"() -> ()  [unwired: 3 in, 1 out]
  n459 = call "4_6_cholesky_decomposition.vi"() -> ()  [unwired: 3 in, 1 out]
  n460 = call "4_5_cholesky_decomposition.vi"() -> ()  [unwired: 3 in, 1 out]
  n461 = call "4_4_cholesky_decomposition.vi"() -> ()  [unwired: 3 in, 1 out]
  n462 = call "4_3_cholesky_decomposition.vi"() -> ()  [unwired: 3 in, 1 out]
  n463 = call "4_2_cholesky_decomposition.vi"() -> ()  [unwired: 3 in, 1 out]
  n464 = call "4_1_cholesky_decomposition.vi"() -> ()  [unwired: 3 in, 1 out]
  n465 = call "3_16_cholesky_decomposition.vi"() -> ()  [unwired: 3 in, 1 out]
  n466 = call "3_15_cholesky_decomposition.vi"() -> ()  [unwired: 3 in, 1 out]
  n467 = call "3_14_cholesky_decomposition.vi"() -> ()  [unwired: 3 in, 1 out]
  n468 = call "3_13_cholesky_decomposition.vi"() -> ()  [unwired: 3 in, 1 out]
  n469 = call "3_12_cholesky_decomposition.vi"() -> ()  [unwired: 3 in, 1 out]
  n470 = call "3_11_cholesky_decomposition.vi"() -> ()  [unwired: 3 in, 1 out]
  n471 = call "3_10_cholesky_decomposition.vi"() -> ()  [unwired: 3 in, 1 out]
  n472 = call "3_9_cholesky_decomposition.vi"() -> ()  [unwired: 3 in, 1 out]
  n473 = call "3_8_cholesky_decomposition.vi"() -> ()  [unwired: 3 in, 1 out]
  n474 = call "3_7_cholesky_decomposition.vi"() -> ()  [unwired: 3 in, 1 out]
  n475 = call "3_6_cholesky_decomposition.vi"() -> ()  [unwired: 3 in, 1 out]
  n476 = call "3_5_cholesky_decomposition.vi"() -> ()  [unwired: 3 in, 1 out]
  n477 = call "3_4_cholesky_decomposition.vi"() -> ()  [unwired: 3 in, 1 out]
  n478 = call "3_3_cholesky_decomposition.vi"() -> ()  [unwired: 3 in, 1 out]
  n479 = call "3_2_cholesky_decomposition.vi"() -> ()  [unwired: 3 in, 1 out]
  n480 = call "3_1_cholesky_decomposition.vi"() -> ()  [unwired: 3 in, 1 out]
  n481 = call "2_16_cholesky_decomposition.vi"() -> ()  [unwired: 3 in, 1 out]
  n482 = call "2_15_cholesky_decomposition.vi"() -> ()  [unwired: 3 in, 1 out]
  n483 = call "2_14_cholesky_decomposition.vi"() -> ()  [unwired: 3 in, 1 out]
  n484 = call "2_13_cholesky_decomposition.vi"() -> ()  [unwired: 3 in, 1 out]
  n485 = call "2_12_cholesky_decomposition.vi"() -> ()  [unwired: 3 in, 1 out]
  n486 = call "2_11_cholesky_decomposition.vi"() -> ()  [unwired: 3 in, 1 out]
  n487 = call "2_10_cholesky_decomposition.vi"() -> ()  [unwired: 3 in, 1 out]
  n488 = call "2_9_cholesky_decomposition.vi"() -> ()  [unwired: 3 in, 1 out]
  n489 = call "2_8_cholesky_decomposition.vi"() -> ()  [unwired: 3 in, 1 out]
  n490 = call "2_7_cholesky_decomposition.vi"() -> ()  [unwired: 3 in, 1 out]
  n491 = call "2_6_cholesky_decomposition.vi"() -> ()  [unwired: 3 in, 1 out]
  n492 = call "2_5_cholesky_decomposition.vi"() -> ()  [unwired: 3 in, 1 out]
  n493 = call "2_4_cholesky_decomposition.vi"() -> ()  [unwired: 3 in, 1 out]
  n494 = call "2_3_cholesky_decomposition.vi"() -> ()  [unwired: 3 in, 1 out]
  n495 = call "2_2_cholesky_decomposition.vi"() -> ()  [unwired: 3 in, 1 out]
  n496 = call "2_1_cholesky_decomposition.vi"() -> ()  [unwired: 3 in, 1 out]
  n497 = call "1_16_cholesky_decomposition.vi"() -> ()  [unwired: 3 in, 1 out]
  n498 = call "1_15_cholesky_decomposition.vi"() -> ()  [unwired: 3 in, 1 out]
  n499 = call "1_14_cholesky_decomposition.vi"() -> ()  [unwired: 3 in, 1 out]
  n500 = call "1_13_cholesky_decomposition.vi"() -> ()  [unwired: 3 in, 1 out]
  n501 = call "1_12_cholesky_decomposition.vi"() -> ()  [unwired: 3 in, 1 out]
  n502 = call "1_11_cholesky_decomposition.vi"() -> ()  [unwired: 3 in, 1 out]
  n503 = call "1_10_cholesky_decomposition.vi"() -> ()  [unwired: 3 in, 1 out]
  n504 = call "1_9_cholesky_decomposition.vi"() -> ()  [unwired: 3 in, 1 out]
  n505 = call "1_8_cholesky_decomposition.vi"() -> ()  [unwired: 3 in, 1 out]
  n506 = call "1_7_cholesky_decomposition.vi"() -> ()  [unwired: 3 in, 1 out]
  n507 = call "1_6_cholesky_decomposition.vi"() -> ()  [unwired: 3 in, 1 out]
  n508 = call "1_5_cholesky_decomposition.vi"() -> ()  [unwired: 3 in, 1 out]
  n509 = call "1_4_cholesky_decomposition.vi"() -> ()  [unwired: 3 in, 1 out]
  n510 = call "1_3_cholesky_decomposition.vi"() -> ()  [unwired: 3 in, 1 out]
  n511 = call "1_2_cholesky_decomposition.vi"() -> ()  [unwired: 3 in, 1 out]
  n512 = call "1_1_cholesky_decomposition.vi"() -> ()  [unwired: 3 in, 1 out]
  n513 = call "cholesky_decomposition_SGL.vi"() -> ()  [unwired: 3 in, 1 out]
